vi "ReadAllCustomKeys.vi"(8 "error in":errorcluster, 11 "Image Reference In":T1) -> (0 "error out":errorcluster, 1 "NumberOfKeys":u32, 2 "Keys":string[](array[string]), 3 "Image Reference Out":T1)   [LabVIEW 2024, in "OpenLvVision_Image.lvlib" / "Management.lvlib"]
doc: "Returns a array of all custom custom data keys associated with the image."
uses:
  Management.lvlib
  TypeDef/Image.ctl
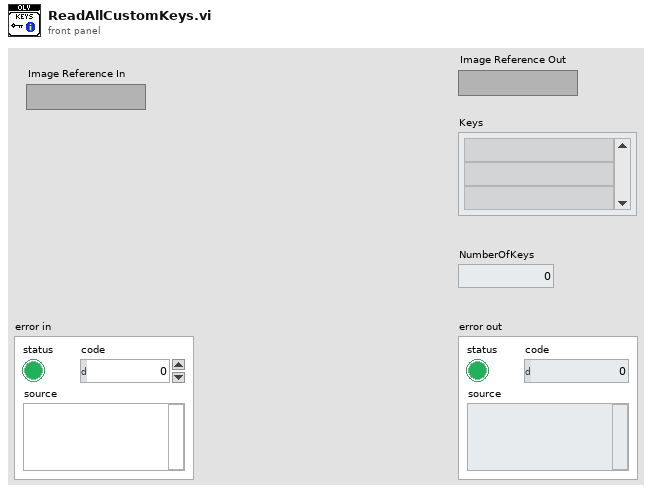
[diagram p1: front panel]
types:
  T1 = typedef "OpenLvVision_Image.lvlib/Management.lvlib/Image.ctl" = refnum<image>
  T2 = typedef "IMAQ Image.ctl" = refnum<image>
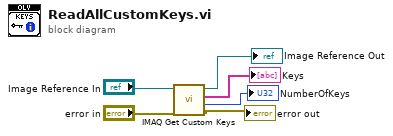
[diagram p0: block diagram]
diagram:
  n1 = call "IMAQ Get Custom Keys"("error in (no error)"="error in", "Image"="Image Reference In") -> ("error out"=→"error out":errorcluster, "Number of Keys"=→"NumberOfKeys":u32, "Keys"=→"Keys":string[], "Image (duplicate)"=→"Image Reference Out":T2)  [unwired: 6 in]
